vi "component_specification_dialog.vi"(4 "default folder path":path, 5 "show label?":bool=TRUE, 6 "show settings?":bool=TRUE, 7 "show configuration?":bool=TRUE, 8 "error in (no error)":errorcluster, 10 "component specification in":T2) -> (0 "error out":errorcluster, 1 "cancelled?":bool, 2 "component specification out":T2)   [LabVIEW 2010]
uses:
  clusters/plugin_specification.ctl
  xcontrols/XComponentSpecification/XComponentSpecification/XComponentSpecification.xctl
panel:
  in  "XComponentSpecification":T1(xcontrol)
  in  "cancel button":bool
  in  "ok button":bool
  # "Component specification"
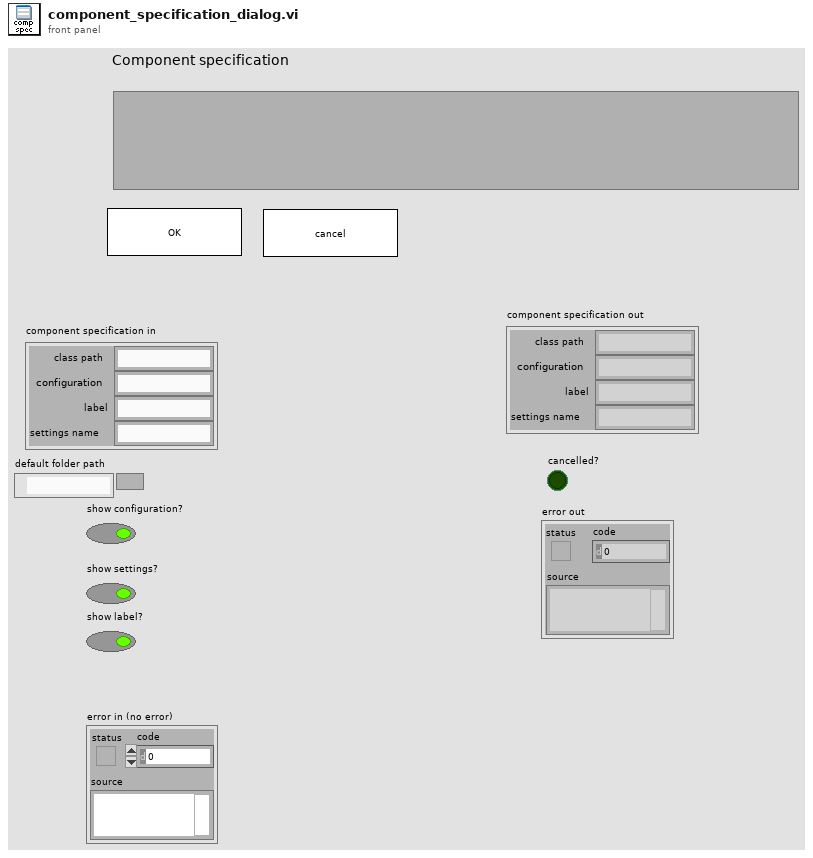
[diagram p1: front panel]
types:
  T1 = cluster{"class path":string, "configuration":string, "label":string, "settings name":string}
  T2 = typedef "plugin_specification.ctl" = cluster{"class path":string, "configuration":string, "label":string, "settings name":string}
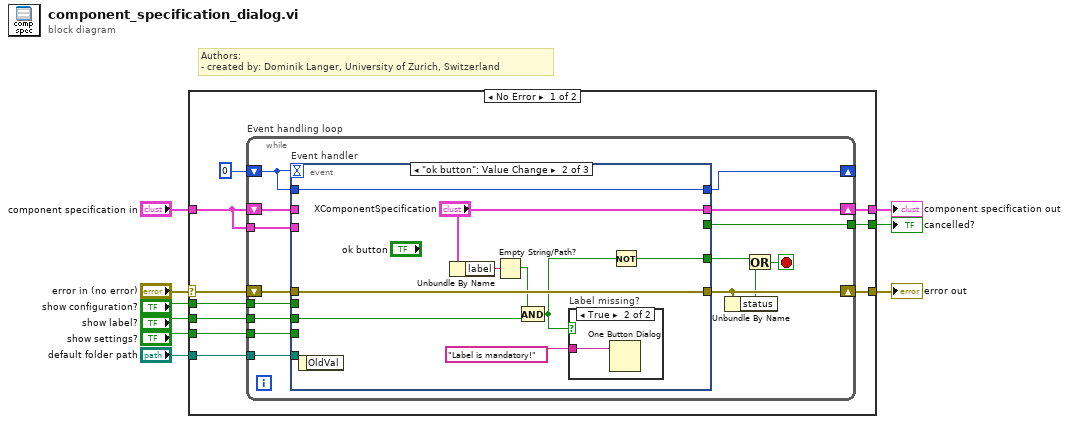
[diagram p0: block diagram]
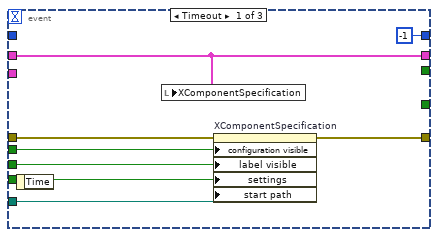
[diagram p2: hidden frame]
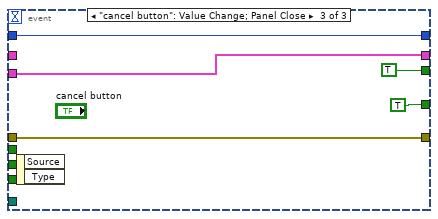
[diagram p4: hidden frame]
diagram:
  # "Authors: \n- created by: Dominik Langer, University of Zurich, Switzerland"
  n1 = case shown="No Error" "error in (no error)" {
    selector: "error in (no error)" -> [w19 w57]
    tunnel: [w18 w57] -> w8
    tunnel: [w14 _] -> w7
    tunnel: "component specification in" -> [w15 _]
    tunnel: [w16 _] -> w5
    tunnel: "default folder path" -> [w13 _]
    tunnel: "show settings?" -> [w12 _]
    tunnel: "show label?" -> [w11 _]
    tunnel: "show configuration?" -> [w10 _]
    frame No Error {
      n2 = while "Event handling loop" {
        shift-right: [w26] -> w18
        shift-left: w19 -> [w34]
        shift-right: [w32] -> _
        shift-left: 0 -> [w33]
        tunnel: [w30] -> w16
        shift-right: [w29] -> w14
        shift-left: w15 -> [w31]
        tunnel: w15 -> [w28]
        tunnel: w13 -> [w27]
        tunnel: w12 -> [w24]
        tunnel: w11 -> [w23]
        tunnel: w10 -> [w22]
        stop <- w25 stop-if-true
        n3 = event "Event handler" shown="[1] \"ok button\": Value Change" {
          selector: _ -> [_ _ _]
          dyn-events: _ -> [_ _ _]
          timeout: w33 -> [_ _ _]
          tunnel: w34 -> [w41 w50 w56]
          tunnel: [w40 w50 w56] -> w26
          tunnel: [_ w44 TRUE] -> w20
          tunnel: w33 -> [_ w49 w54]
          tunnel: [-1 w49 w54] -> w32
          tunnel: w31 -> [w39 _ _]
          tunnel: [_ _ TRUE] -> w30
          tunnel: [w39 "XComponentSpecification" w52] -> w29
          tunnel: w28 -> [_ _ w52]
          tunnel: w27 -> [w38 _ _]
          tunnel: w24 -> [w37 _ _]
          tunnel: w23 -> [w36 w46 _]
          tunnel: w22 -> [w35 _ _]
          event Timeout {
            n4 = event-data() -> ()  [unwired: 2 out]
            n5 = local write "XComponentSpecification"(w39) -> ()
            n6 = property on="XComponentSpecification" class="XComponentSpecification (strict"(error in=w41, "configuration visible"=w35, "label visible"=w36, "settings"=w37, "start path"=w38) -> (error out=w40:errorcluster)  [unwired: 1 in, 1 out]
          }
          event "ok button": Value Change {
            n7 = event-data() -> ()  [unwired: 2 out]
            n8 = Unbundle By Name("XComponentSpecification") -> ("label"=w47:string)
            n9 = Empty String/Path?(string/path=w47) -> (empty?=w43:bool)
            n10 = And(x=w43, y=w46) -> ()  [unwired: 1 out]
            n11 = case "Label missing?" shown="True" w43 {
              tunnel: "Label is mandatory!" -> [_ w51]
              frame False {
              }
              frame True {
                n12 = One Button Dialog(message=w51) -> ()  [unwired: 1 in, 1 out]
              }
            }
            n13 = Not(x=w43) -> (.not. x?=w44:bool)
          }
          event "cancel button": Value Change; Panel Close {
            n14 = event-data() -> ()  [unwired: 3 out]
          }
        }
        n15 = Unbundle By Name(w26) -> ("status"=w21:bool)
        n16 = Or(x=w20, y=w21) -> (x .or. y?=w25:bool)
      }
    }
    frame Error {
    }
  }
  "error out" <- w8
  "component specification out" <- w7
  "cancelled?" <- w5
